vi "dynamic.vi"(8 "error in (no error)":errorcluster, 11 "parent in":refnum<class "Parent.lvclass">) -> (0 "error out":errorcluster, 2 "message":string="Parent Dynamic VI", 3 "parent out":refnum<class "Parent.lvclass">)   [LabVIEW 2021, in "Parent.lvclass"]
uses:
  Parent.lvclass
  Parent.lvclass/Parent.ctl
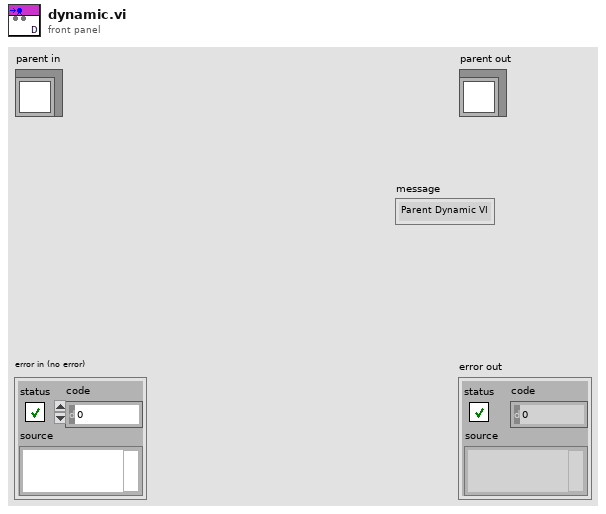
[diagram p1: front panel]
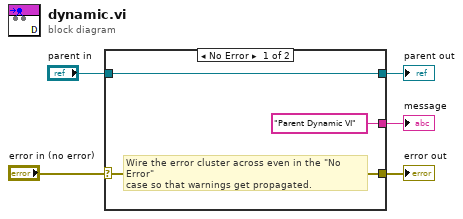
[diagram p0: block diagram]
diagram:
  n1 = case shown="No Error" "error in (no error)" {
    selector: "error in (no error)" -> [w7 w10]
    tunnel: [w7 w10] -> w4
    tunnel: [w8 w9] -> w2
    tunnel: "parent in" -> [w8 w9]
    tunnel: ["Parent Dynamic VI" ("message") _] -> w1
    frame No Error {
      # "Wire the error cluster across even in the \"No Error\"\ncase so that warnings get propagated."
    }
    frame Error {
    }
  }
  "error out" <- w4
  "parent out" <- w2
  "message" <- w1
